vi "GT Init Look Ahead.vi"(0 "cardNum":i16, 1 "accMax":dbl, 2 "pLookAheadBuf":T1(array[cluster]), 5 "crd":i16, 7 "fifo":i16, 9 "T":dbl, 11 "error in (no error)":errorcluster caption="错误输入（无错误）", 12 "n":i16) -> (4 "pLookAheadBuf out":T1(array[cluster]), 6 "function return":i16, 15 "error out":errorcluster caption="错误输出")   [LabVIEW 2020, in "gts.lvlib"]
doc: "GT_API GT_InitLookAhead(short cardNum,short crd,short fifo,double T,double accMax,short n,TCrdData *pLookAheadBuf);"
uses:
  gts.lvlib
  dll/32bit/multi_card/gts.dll
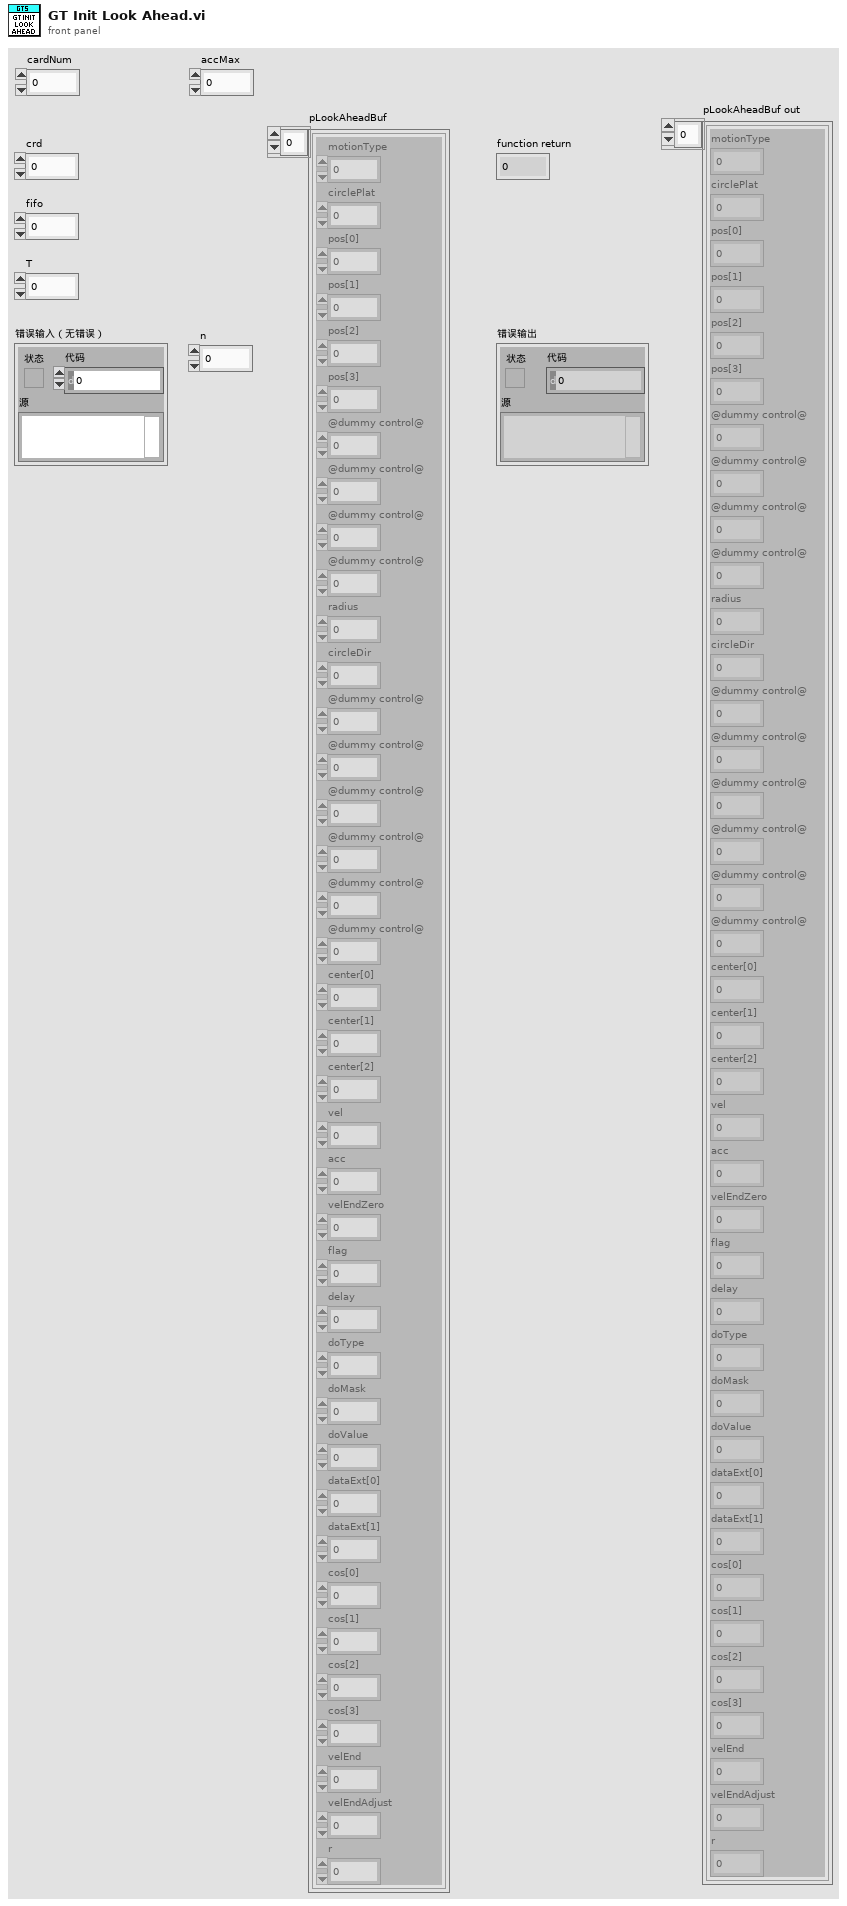
[diagram p1: front panel]
types:
  T1 = cluster{"motionType":i16, "circlePlat":i16, "pos[0]":i32, "pos[1]":i32, "pos[2]":i32, "pos[3]":i32, "@dummy control@":i8, "@dummy control@":i8, "@dummy control@":i8, "@dummy control@":i8, "radius":dbl, "circleDir":i16, "@dummy control@":i8, "@dummy control@":i8, "@dummy control@":i8, "@dummy control@":i8, "@dummy control@":i8, "@dummy control@":i8, "center[0]":dbl, "center[1]":dbl, "center[2]":dbl, "vel":dbl, "acc":dbl, "velEndZero":i16, "flag":i16, "delay":u16, "doType":i16, "doMask":u16, "doValue":u16, "dataExt[0]":u16, "dataExt[1]":u16, "cos[0]":dbl, "cos[1]":dbl, "cos[2]":dbl, "cos[3]":dbl, "velEnd":dbl, "velEndAdjust":dbl, "r":dbl}[]
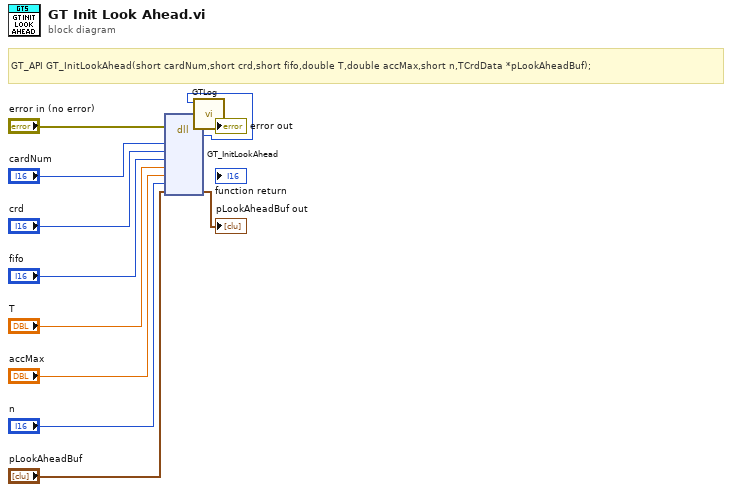
[diagram p0: block diagram]
diagram:
  # "GT_API GT_InitLookAhead(short cardNum,short crd,short fifo,double T,double accMax,short n,TCrdData *pLookAheadBuf);"
  n1 = dll-call lib="C:/1228/dll/32bit/multi_card/gts.dll" fn="GT_InitLookAhead"(error in="error in (no error)", "cardNum"="cardNum", "crd"="crd", "fifo"="fifo", "T"="T", "accMax"="accMax", "n"="n", "pLookAheadBuf"="pLookAheadBuf") -> (error out=w3:errorcluster, "返回类型"=w1:i16, "pLookAheadBuf"=→"pLookAheadBuf out":T1)  [unwired: 8 in, 1 out]
  n2 = call "GTLog.vi"("error in (no error)"=w3, "Numeric"=w1) -> ("error out"=→"error out":errorcluster)  [unwired: 9 in]
